vi "Apply Filter Mask.vi"(8 "error in (no error)":errorcluster, 10 "Filter Mask":bool[][](array[boolean]), 11 "2DArrayManager in":refnum<class "2DArrayManager.lvclass">) -> (0 "error out":errorcluster, 3 "2DArrayManager out":refnum<class "2DArrayManager.lvclass">)   [LabVIEW 2020, in "OOPanel.lvlib" / "2DArrayManager.lvclass"]
uses:
  2DArrayManager.lvclass
  2D Position.ctl
  OOPanel.lvlib
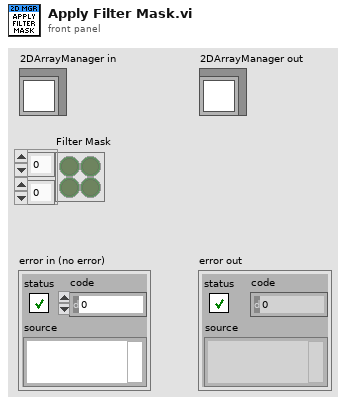
[diagram p1: front panel]
types:
  T1 = typedef "OOPanel.lvlib/2D Position.ctl" = cluster{"H":i32, "V":i32}
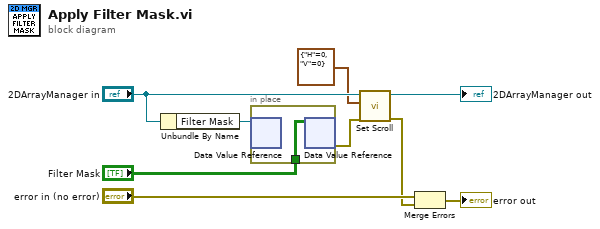
[diagram p0: block diagram]
diagram:
  n1 = Unbundle By Name("2DArrayManager in") -> ("Filter Mask"=w8:refnum<data-value>)
  n2 = in-place {
    in-place-border: "Filter Mask" -> [w10]
    n3 = in-place-dvr #1(w8) -> ()  [unwired: 2 out]
    n4 = in-place-dvr #1(w10) -> (w2:errorcluster)  [unwired: 1 out]
  }
  n5 = call "Set Scroll.vi"("error in (no error)"=w2, "Position"=T1 {"H"=0, "V"=0}, "2DArrayManager in"="2DArrayManager in") -> ("error out"=w1:errorcluster, "2DArrayManager out"=→"2DArrayManager out":refnum<class "2DArrayManager.lvclass">)  [unwired: 7 in]
  n6 = Merge Errors("error in (no error)", w1) -> (→"error out":errorcluster)
